vi "REWORK_get_operations_and_results.vi"(6 "executed_SQL_statement_in":string, 8 "error_in":errorcluster, 11 "SQL_result":variant) -> (0 "error_out":errorcluster, 4 "executed_SQL_statement_out":string)   [LabVIEW 2019]
uses:
  FGV/REWORK_records_display/FGV_REWORK_records_display.ctl
  FGV/REWORK_destination_selector/FGV_REWORK_destination_selector.ctl
  FGV/SQL_connection/FGV_REWORK_SQL_connection.ctl
  _misc/AULocalize/SubVIs/Get Localized Phrase Compact Interface 0D.vi
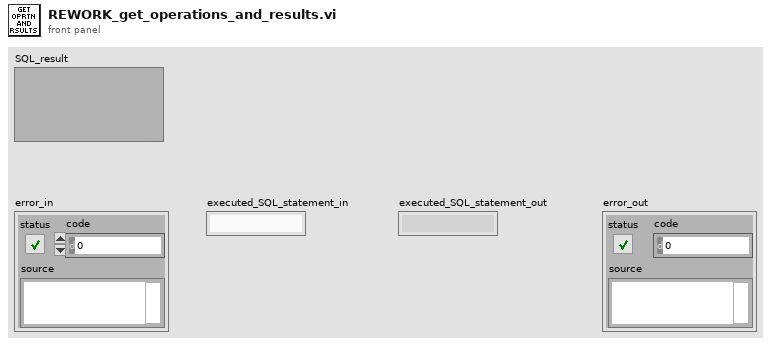
[diagram p1: front panel]
types:
  T1 = typedef "FGV_REWORK_SQL_connection.ctl" = enum16{"initialize", "connect", "read_tables", "read_columns", "SELECT", "INSERT", "UPDATE", "DELETE", "EXEC + headers", "EXEC", "TRANSACTION", "connection_active?", "disconnect"}
  T2 = typedef "FGV_REWORK_destination_selector.ctl" = enum16{"initialize", "set_values", "display_values", "set_new_login", "enable", "disable", "disable_gray", "get_rework_to", "clear"}
  T3 = typedef "FGV_REWORK_records_display.ctl" = enum16{"initialize", "set_serial", "set_header", "set_operations", "set_results", "set_batches", "get_serial", "get_part_ID", "get_operation_IDs", "toggle_results", "show_all_results", "hide_all_results", "display", "clear"}
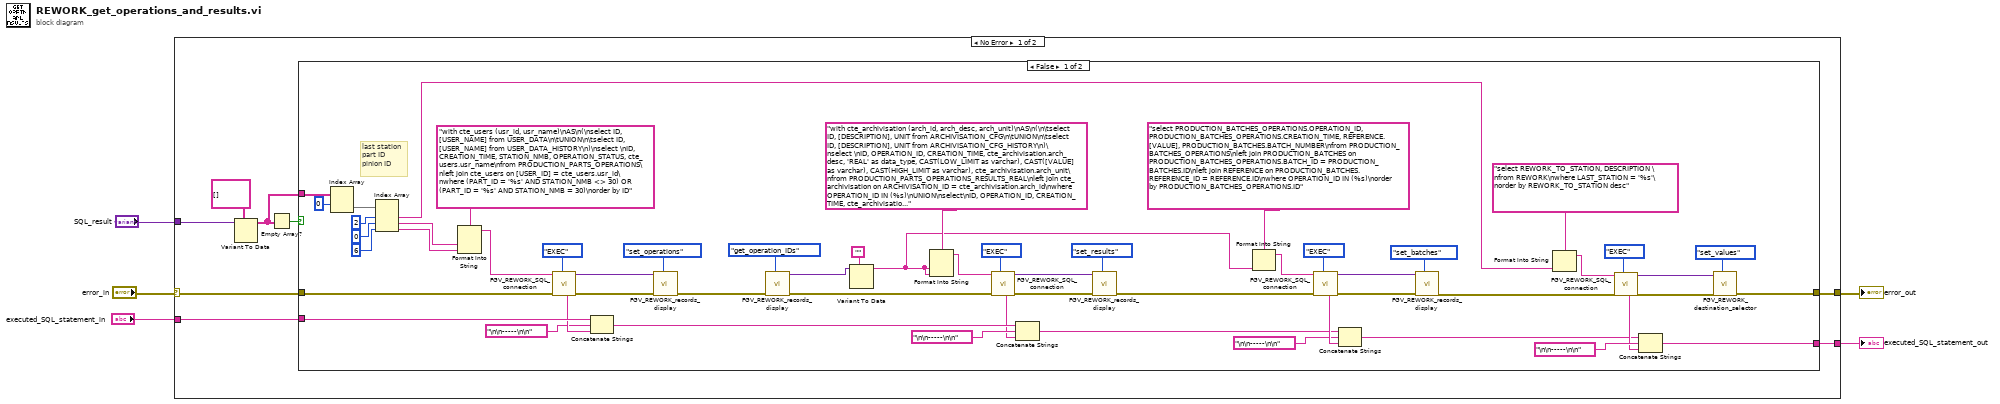
[diagram p0: block diagram]
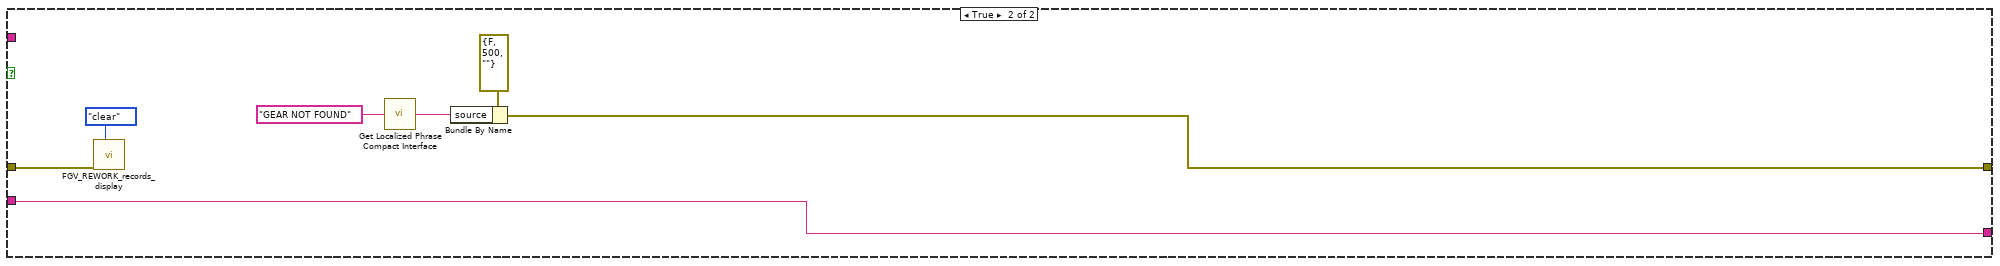
[diagram p2: hidden frame]
diagram:
  n1 = case shown="No Error" "error_in" {
    selector: "error_in" -> [w10 w78]
    tunnel: [w13 w77] -> w5
    tunnel: "executed_SQL_statement_in" -> [w12 w77]
    tunnel: [w11 w78] -> w3
    tunnel: "SQL_result" -> [w9 _]
    frame No Error {
      n2 = Variant To Data(type=string[][] [], Variant=w9) -> (data=w7:string[][])  [unwired: 1 in, 1 out]
      n3 = Empty Array?(array=w7) -> (empty?=w8:bool)
      n4 = case shown="False" w8 {
        tunnel: w10 -> [w69 w74]
        tunnel: [w26 w72] -> w11
        tunnel: w12 -> [w55 w76]
        tunnel: [w15 w76] -> w13
        tunnel: w7 -> [w64 _]
        frame False {
          # "last station\npart ID\npinion ID"
          n5 = Index Array(array=w64, index (row)=0) -> (element=w62:string[])  [unwired: 1 in]
          n6 = Index Array(array=w62, index #1=2 ("index"), index #2=0 ("index"), index #3=6 ("index")) -> (element #1=w14:string, element #2=w57:string, element #3=w56:string)
          n7 = Format Into String(format string="with cte_users (usr_id, usr_name)\nAS\n(\nselect ID, [USER_NAME] from USER_DATA\n\tUNION\n\tselect ID, [USER_NAME] from USER_DATA_HISTORY\n)\nselect \nID, CREATION_TIME, STATION_NMB, OPERATION_STATUS, cte_users.usr_name\nfrom PRODUCTION_PARTS_OPERATIONS\nleft join cte_users on [USER_ID] = cte_users.usr_id\nwhere (PART_ID = '%s' AND STATION_NMB <> 30) OR (PART_ID = '%s' AND STATION_NMB = 30)\norder by ID", w57, w56) -> (resulting string=w59:string)  [unwired: 2 in, 1 out]
          n8 = call "FGV_REWORK_SQL_connection.vi"("options"=FGV_REWORK_SQL_connection."EXEC", "error_in"=w69, "SQL_statement"=w59) -> ("error_out"=w66:errorcluster, "SQL_result"=w65:variant, "executed_SQL_statement"=w54:string)  [unwired: 4 in, 2 out]
          n9 = Concatenate Strings(w55, "\n\n-----\n\n" ("string"), w54) -> (w47:string)
          n10 = call "FGV_REWORK_records_display.vi"("options"=FGV_REWORK_records_display."set_operations", "error_in"=w66, "input"=w65) -> ("error_out"=w43:errorcluster)  [unwired: 7 in, 1 out]
          n11 = call "FGV_REWORK_records_display.vi"("options"=FGV_REWORK_records_display."get_operation_IDs", "error_in"=w43) -> ("error_out"=w42:errorcluster, "output"=w40:variant)  [unwired: 8 in]
          n12 = Variant To Data(type="", Variant=w40) -> (data=w28:string)  [unwired: 1 in, 1 out]
          n13 = Format Into String(format string="with cte_archivisation (arch_id, arch_desc, arch_unit)\nAS\n(\n\tselect ID, [DESCRIPTION], UNIT from ARCHIVISATION_CFG\n\tUNION\n\tselect ID, [DESCRIPTION], UNIT from ARCHIVISATION_CFG_HISTORY\n)\nselect \nID, OPERATION_ID, CREATION_TIME, cte_archivisation.arch_desc, 'REAL' as data_type, CAST(LOW_LIMIT as varchar), CAST([VALUE] as varchar), CAST(HIGH_LIMIT as varchar), cte_archivisation.arch_unit\nfrom PRODUCTION_PARTS_OPERATIONS_RESULTS_REAL\nleft join cte_archivisation on ARCHIVISATION_ID = cte_archivisation.arch_id\nwhere OPERATION_ID IN (%s)\nUNION\nselect\nID, OPERATION_ID, CREATION_TIME, cte_archivisation.arch_desc, 'STRING' as data_type, '-', [VALUE], '-', cte_archivisation.arch_unit\nfrom PRODUCTION_PARTS_OPERATIONS_RESULTS_STRING\nleft join cte_archivisation on ARCHIVISATION_ID = cte_archivisation.arch_id\nwhere OPERATION_ID IN (%s)\norder by data_type, ID", w28, w28) -> (resulting string=w45:string)  [unwired: 2 in, 1 out]
          n14 = call "FGV_REWORK_SQL_connection.vi"("options"=FGV_REWORK_SQL_connection."EXEC", "error_in"=w42, "SQL_statement"=w45) -> ("error_out"=w50:errorcluster, "SQL_result"=w52:variant, "executed_SQL_statement"=w46:string)  [unwired: 4 in, 2 out]
          n15 = Concatenate Strings(w47, "\n\n-----\n\n" ("string"), w46) -> (w29:string)
          n16 = call "FGV_REWORK_records_display.vi"("options"=FGV_REWORK_records_display."set_results", "error_in"=w50, "input"=w52) -> ("error_out"=w30:errorcluster)  [unwired: 7 in, 1 out]
          n17 = Format Into String(format string="select PRODUCTION_BATCHES_OPERATIONS.OPERATION_ID, PRODUCTION_BATCHES_OPERATIONS.CREATION_TIME, REFERENCE.[VALUE], PRODUCTION_BATCHES.BATCH_NUMBER\nfrom PRODUCTION_BATCHES_OPERATIONS\nleft join PRODUCTION_BATCHES on PRODUCTION_BATCHES_OPERATIONS.BATCH_ID = PRODUCTION_BATCHES.ID\nleft join REFERENCE on PRODUCTION_BATCHES.REFERENCE_ID = REFERENCE.ID\nwhere OPERATION_ID IN (%s)\norder by PRODUCTION_BATCHES_OPERATIONS.ID", w28) -> (resulting string=w37:string)  [unwired: 2 in, 1 out]
          n18 = call "FGV_REWORK_SQL_connection.vi"("options"=FGV_REWORK_SQL_connection."EXEC", "error_in"=w30, "SQL_statement"=w37) -> ("error_out"=w33:errorcluster, "SQL_result"=w31:variant, "executed_SQL_statement"=w36:string)  [unwired: 4 in, 2 out]
          n19 = Concatenate Strings(w29, "\n\n-----\n\n" ("string"), w36) -> (w16:string)
          n20 = call "FGV_REWORK_records_display.vi"("options"=FGV_REWORK_records_display."set_batches", "error_in"=w33, "input"=w31) -> ("error_out"=w19:errorcluster)  [unwired: 7 in, 1 out]
          n21 = Format Into String(format string="select REWORK_TO_STATION, DESCRIPTION \nfrom REWORK\nwhere LAST_STATION = '%s'\norder by REWORK_TO_STATION desc", w14) -> (resulting string=w21:string)  [unwired: 2 in, 1 out]
          n22 = call "FGV_REWORK_SQL_connection.vi"("options"=FGV_REWORK_SQL_connection."EXEC", "error_in"=w19, "SQL_statement"=w21) -> ("error_out"=w18:errorcluster, "SQL_result"=w17:variant, "executed_SQL_statement"=w22:string)  [unwired: 4 in, 2 out]
          n23 = Concatenate Strings(w16, "\n\n-----\n\n" ("string"), w22) -> (w15:string)
          n24 = call "FGV_REWORK_destination_selector.vi"("options"=FGV_REWORK_destination_selector."set_values", "error_in"=w18, "input"=w17) -> ("error_out"=w26:errorcluster)  [unwired: 7 in, 1 out]
        }
        frame True {
          n25 = call "FGV_REWORK_records_display.vi"("options"=FGV_REWORK_records_display."clear", "error_in"=w74) -> ()  [unwired: 8 in, 2 out]
          n26 = call-poly "Get Localized Phrase Compact Interface.vi"("Key"="GEAR NOT FOUND" ("source")) -> ("Translated Phrase"=w71:string)
          n27 = Bundle By Name(cluster=errorcluster {"status"=FALSE, "code"=500, "source"=""} ("error IO"), "source"=w71) -> (w72:errorcluster)
        }
      }
    }
    frame Error {
    }
  }
  "executed_SQL_statement_out" <- w5
  "error_out" <- w3
